vi "WaveformSubset.vi"(8 "error in (no error)":errorcluster, 9 "t2 (s)":dbl, 10 "t1 (s)":dbl, 11 "wfm in":waveform(dbl)) -> (0 "error out":errorcluster, 3 "wfm out":waveform(dbl))   [LabVIEW 2025]
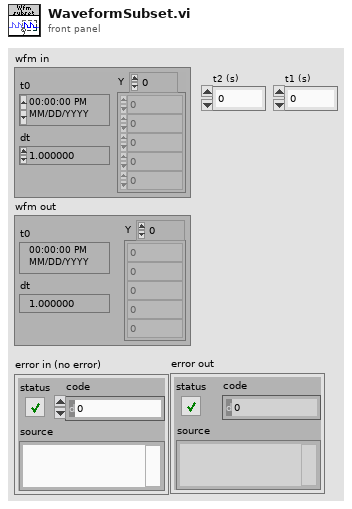
[diagram p1: front panel]
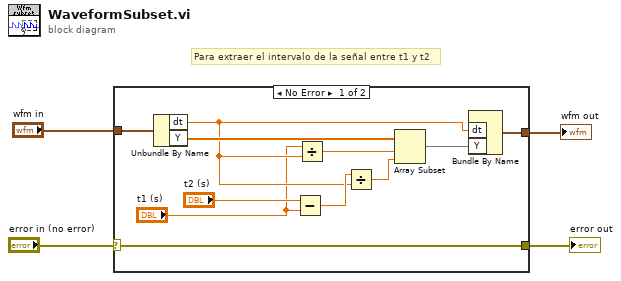
[diagram p0: block diagram]
diagram:
  # "Para extraer el intervalo de la señal entre t1 y t2"
  n1 = case shown="No Error" "error in (no error)" {
    selector: "error in (no error)" -> [w14 w16]
    tunnel: [w14 w16] -> w3
    tunnel: "wfm in" -> [w13 w17]
    tunnel: [w7 w17] -> w1
    frame No Error {
      n2 = Unbundle By Name(w13) -> ("dt"=w8:dbl, "Y"=w15:dbl[])
      n3 = Subtract(x="t2 (s)", y="t1 (s)") -> (x-y=w11:dbl)
      n4 = Divide(x="t1 (s)", y=w8) -> (x/y=w12:dbl)
      n5 = Divide(x=w11, y=w8) -> (x/y=w10:dbl)
      n6 = Array Subset(array=w15, index=w12, length=w10) -> (w9:dbl[])
      n7 = Bundle By Name("dt"=w8, "Y"=w9) -> (w7:waveform(dbl))  [unwired: 1 in]
    }
    frame Error {
    }
  }
  "error out" <- w3
  "wfm out" <- w1
